vi "get time stamp.vi"(8 "error in (no error)":errorcluster, 11 "Point Grey Camera in":refnum<class "Point Grey Camera.lvclass">) -> (0 "error out":errorcluster, 3 "Point Grey Camera out":refnum<class "Point Grey Camera.lvclass">)   [LabVIEW 2020, in "Point Grey Camera.lvclass"]
uses:
  Point Grey Camera.lvclass
  Point Grey Camera.lvclass/Point Grey Camera.ctl
panel:
  out "timestamp":dbl
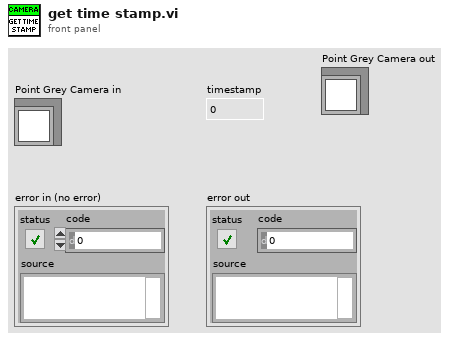
[diagram p1: front panel]
types:
  T1 = typedef "IMAQ Image.ctl" = refnum<image>
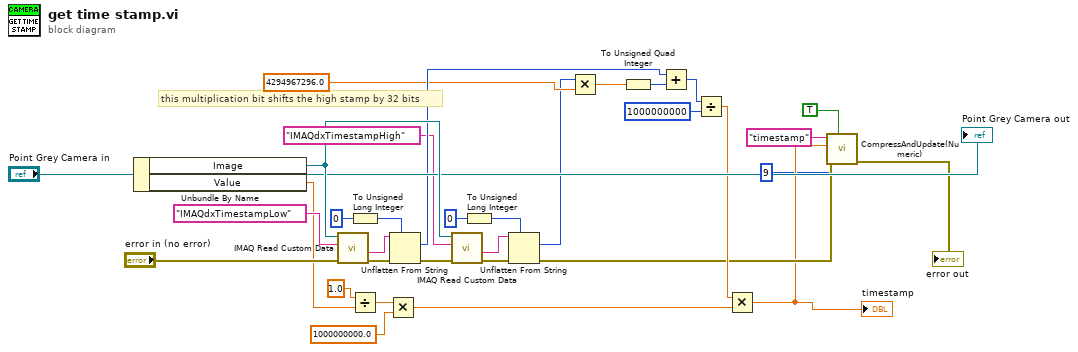
[diagram p0: block diagram]
diagram:
  # "this multiplication bit shifts the high stamp by 32 bits"
  n1 = Unbundle By Name("Point Grey Camera in") -> ("Image"=w29:T1, "Value"=w10:dbl)
  n2 = call "IMAQ Read Custom Data"("error in (no error)"="error in (no error)", "Key"="IMAQdxTimestampLow", "Image"=w29) -> ("error out"=w32:errorcluster, "Custom Data Out"=w16:string)  [unwired: 6 in, 1 out]
  n3 = To Unsigned Long Integer(number=u32 0) -> (unsigned 32bit integer=w15:u32)
  n4 = Divide(x=1.0, y=w10) -> (x/y=w9:dbl)
  n5 = Multiply(x=w9, y=1000000000.0) -> (x*y=w7:dbl)
  n6 = Unflatten From String(type=w15, binary string=w16, error in (no error)=w32) -> (value=w23:u32, error out=w33:errorcluster)  [unwired: 2 in, 1 out]
  n7 = call "IMAQ Read Custom Data"("error in (no error)"=w33, "Key"="IMAQdxTimestampHigh", "Image"=w29) -> ("error out"=w31:errorcluster, "Custom Data Out"=w19:string)  [unwired: 6 in, 1 out]
  n8 = To Unsigned Long Integer(number=u32 0) -> (unsigned 32bit integer=w18:u32)
  n9 = Unflatten From String(type=w18, binary string=w19, error in (no error)=w31) -> (value=w20:u32, error out=w6:errorcluster)  [unwired: 2 in, 1 out]
  n10 = Multiply(x=w20, y=4294967296.0) -> (x*y=w22:dbl)
  n11 = To Unsigned Quad Integer(1:w22) -> (0:w24:u64)
  n12 = Add(x=w23, y=w24) -> (x+y=w25:u64)
  n13 = Divide(x=w25, y=u64 1000000000) -> (x/y=w27:dbl)
  n14 = Multiply(x=w27, y=w7) -> (x*y=w3:dbl)
  "timestamp" <- w3
  n15 = call "CompressAndUpdate(Numeric).vi"("force CVT update (false)"=TRUE, "error in"=w6, "precision (6)"=i16 9, "Numeric"=w3, "command or variable name"="timestamp") -> ("error out"=→"error out":errorcluster)  [unwired: 6 in]
  "Point Grey Camera out" <- "Point Grey Camera in"
